vi "voltSet.vi"() -> ()   [LabVIEW 2016]
uses:
  i2c/VIs/ControlI2C.lvlib
panel:
  in  "stop":bool
  in  "OK Button":bool
  out "Boolean":bool
  in  "voltage":dbl
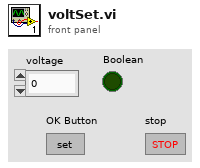
[diagram p1: front panel]
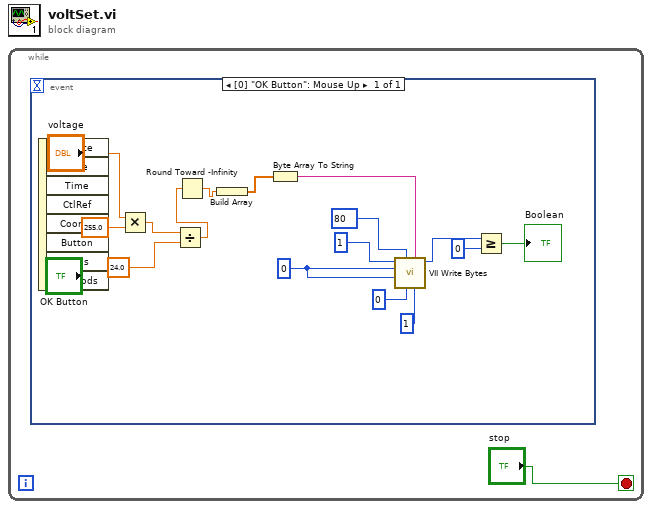
[diagram p0: block diagram]
diagram:
  n1 = while {
    stop <- "stop" stop-if-true
    n2 = event shown="[0] \"OK Button\": Mouse Up" {
      selector: _ -> [_]
      dyn-events: _ -> [_]
      timeout: _ -> [_]
      event "OK Button": Mouse Up {
        w7 = 0 ("DevIndex")
        n3 = event-data() -> ()  [unwired: 1 in, 8 out]
        n4 = Multiply(x="voltage", y=255.0) -> (x*y=w15:dbl)
        n5 = Divide(x=w15, y=24.0) -> (x/y=w13:dbl)
        n6 = Round Toward -Infinity(1:w13) -> (0:w12:dbl)
        n7 = Build Array(w12) -> (w11:dbl[])
        n8 = Byte Array To String(unsigned byte array=w11) -> (string=w9:string)
        n9 = call "VII Write Bytes.vi"("Len"=u16 1, "pWriteData"=w9, "SubAddr"=0, "SlaveAddr"=u16 80, "I2CIndex"=w7, "DevIndex"=w7, "DevType"=1) -> ("function return"=w4:i32)  [unwired: 3 in, 1 out]
        n10 = Greater Or Equal?(x=w4, y=0) -> (x >= y?=→"Boolean":bool)
      }
    }
  }
